vi "MAIN.vi"() -> ()   [LabVIEW 2016, in "副屏.lvlib"]
uses:
  <vilib>/Utility/miscctls.llb/LVPointTypeDef.ctl
  PLC/PLC.lvlib
  <vilib>/Utility/config.llb/NI_LVConfig.lvlib
panel:
  out "单位":string
  out "测试浓度":string
  out "英文标题":string
  out "中文标题":string
  out "公司名称":string
  out "时间":string="2018"
  out "日":string="12"
  out "月":string="12"
  out "年":string="2018"
  # "年"
  # "月"
  # "日"
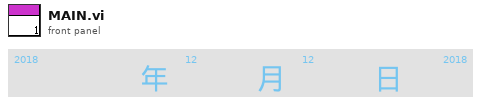
[diagram p1: front panel]
types:
  T1 = cluster{"显示参数中文名":string, "显示参数英文名":string, "显示浓度":string, "显示单位":string}
  T2 = typedef "LVPointTypeDef.ctl" = cluster{"Horizontal":i16, "Vertical":i16}
  T3 = typedef "NI_LVConfig.lvlib/Config Data RefNum.ctl" = refnum<k1>
  T4 = cluster{"AD0":sgl, "AD1":sgl, "AD2":sgl, "AD3":sgl, "AD4":sgl, "AD5":sgl}
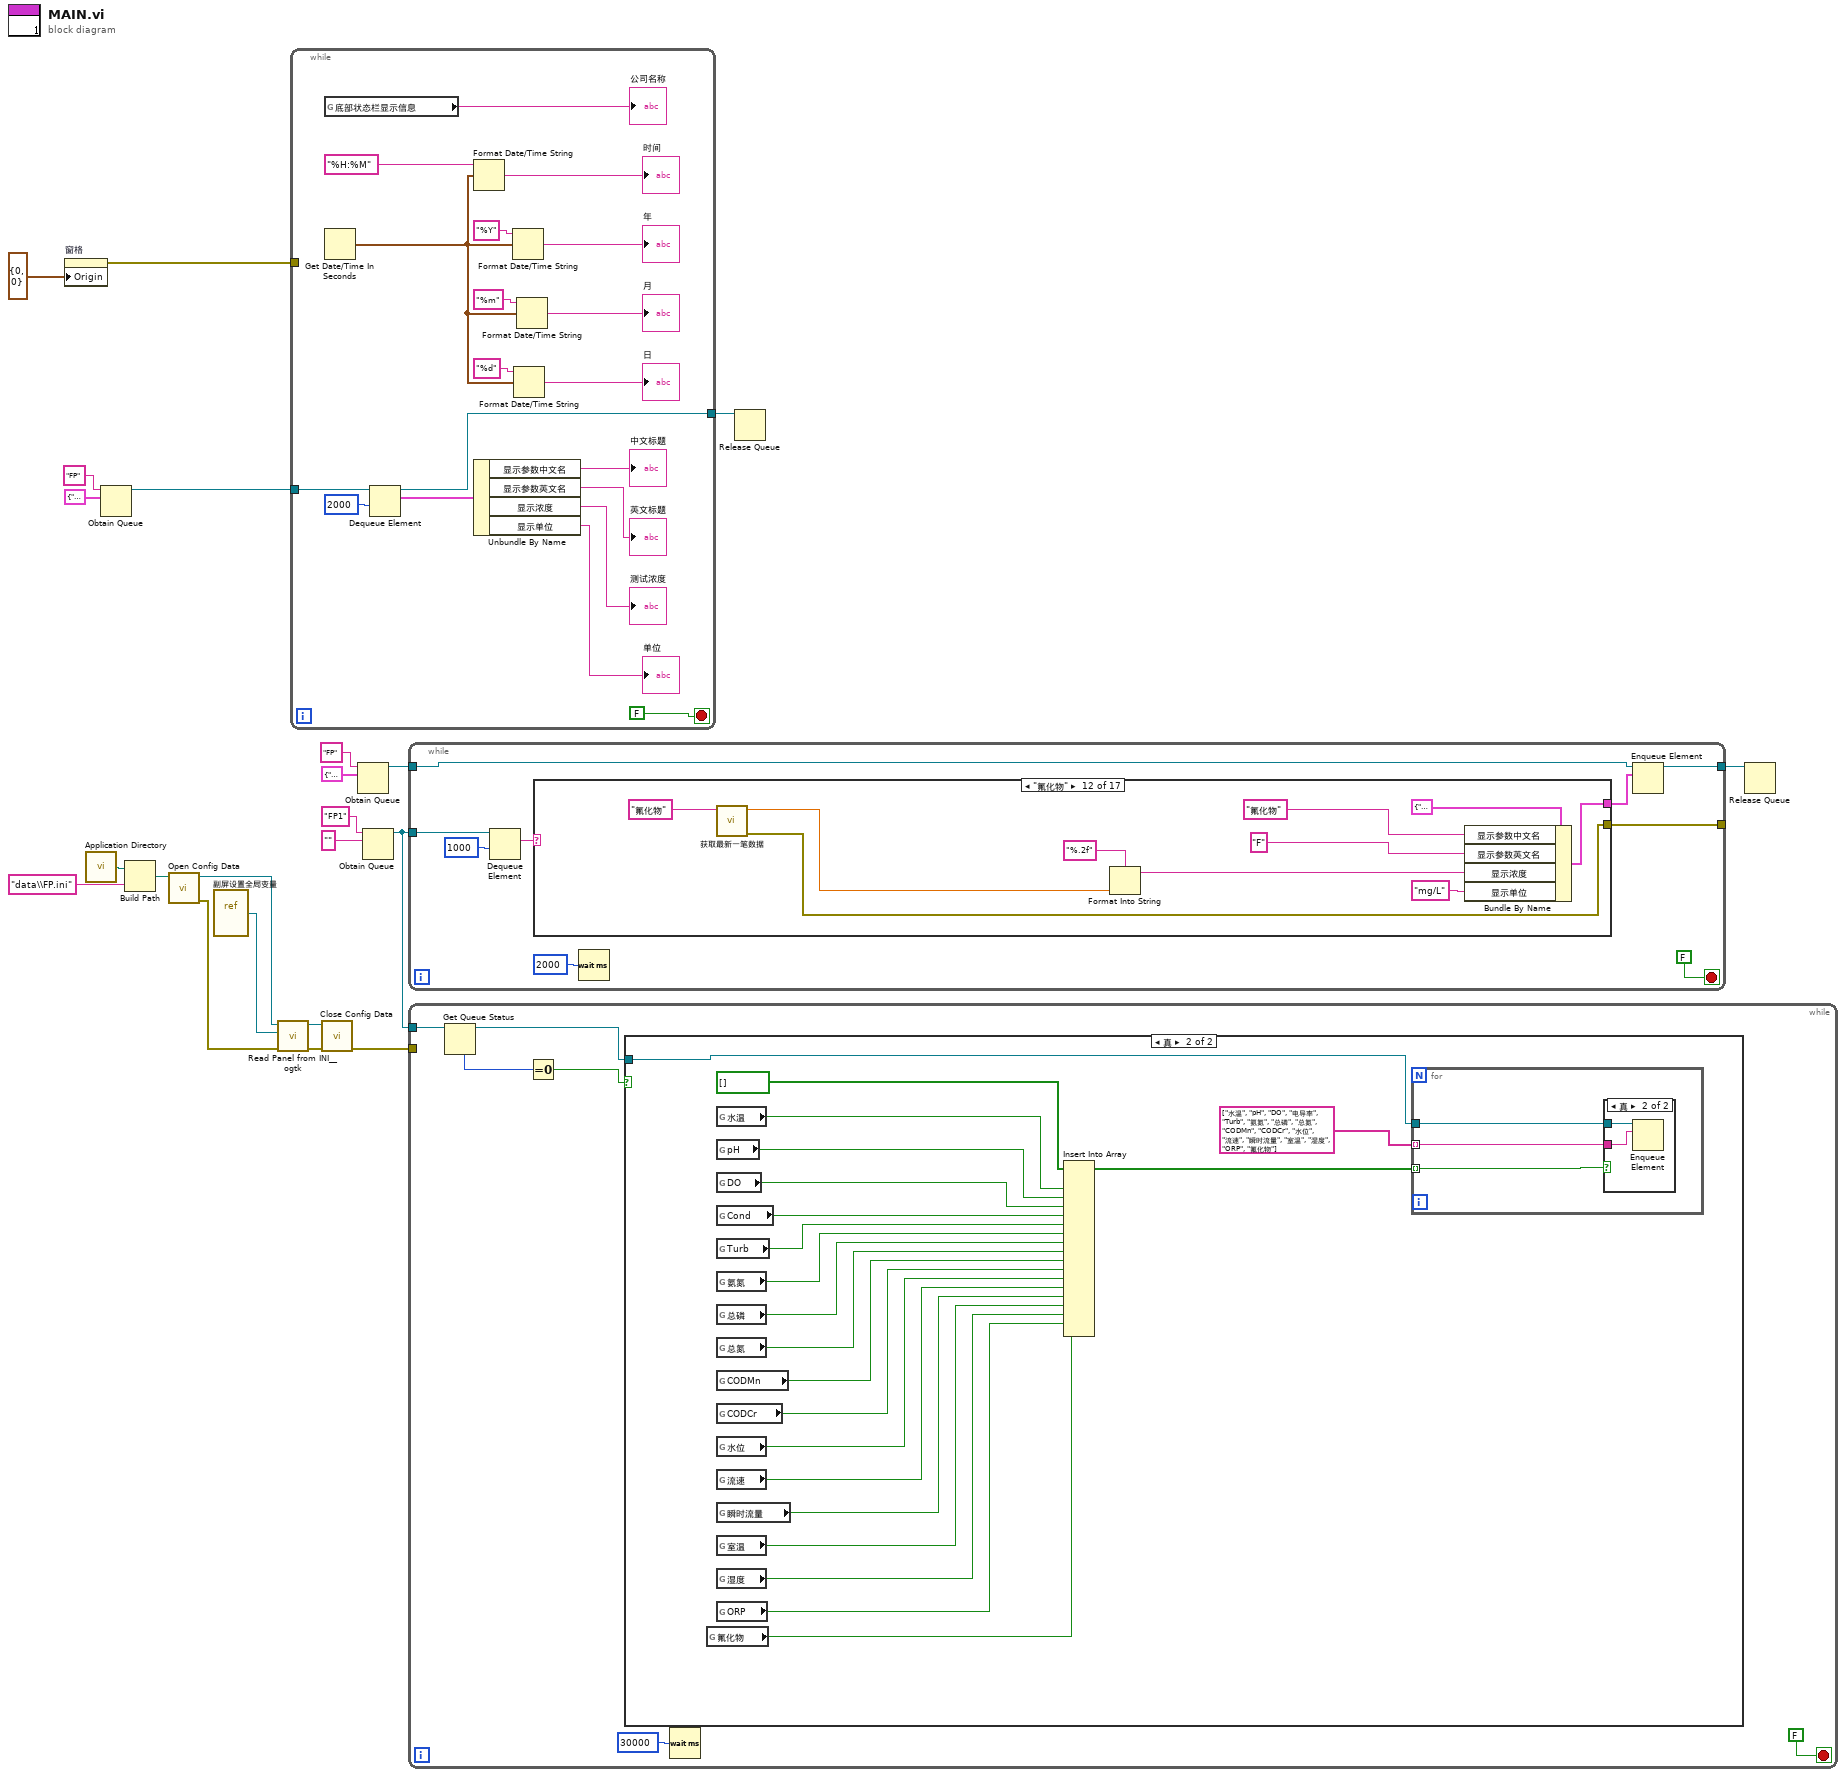
[diagram p0: block diagram]
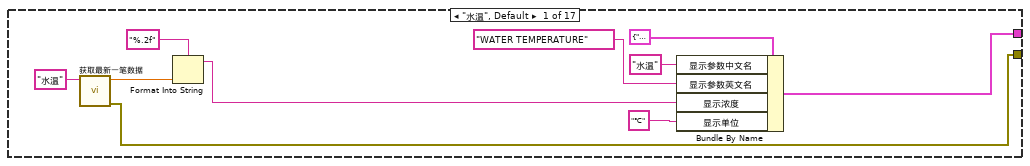
[diagram p4: hidden frame]
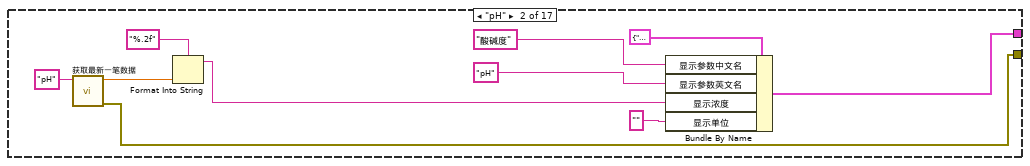
[diagram p5: hidden frame]
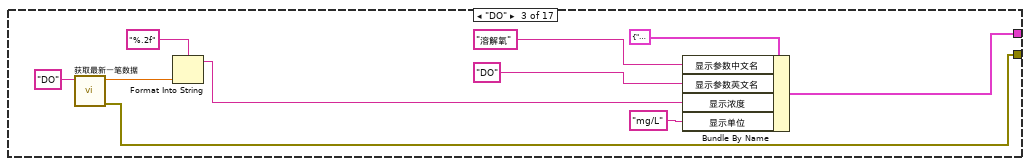
[diagram p6: hidden frame]
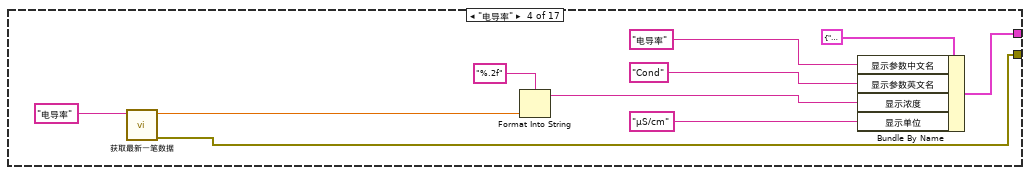
[diagram p7: hidden frame]
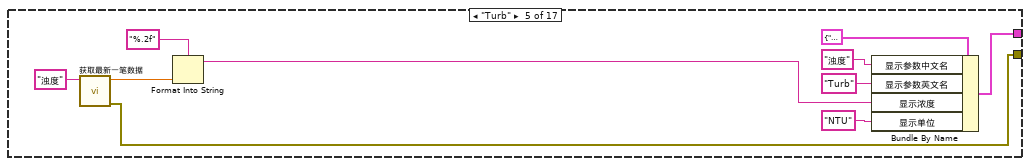
[diagram p8: hidden frame]
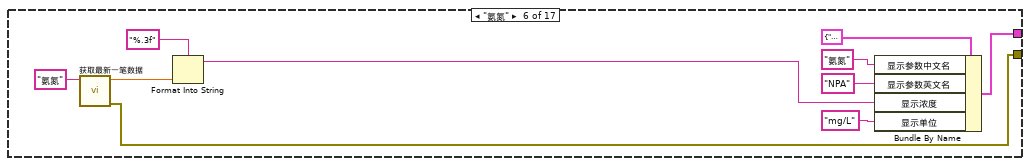
[diagram p9: hidden frame]
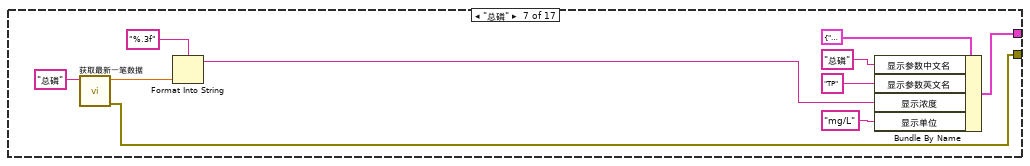
[diagram p10: hidden frame]
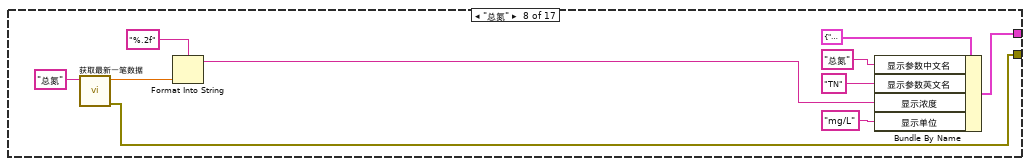
[diagram p11: hidden frame]
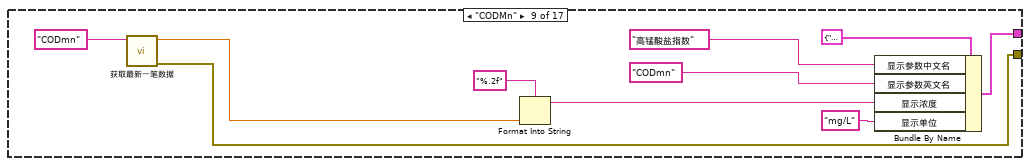
[diagram p12: hidden frame]
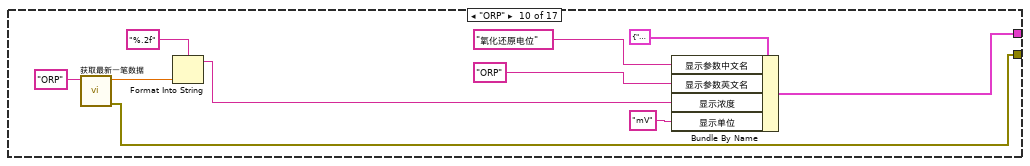
[diagram p13: hidden frame]
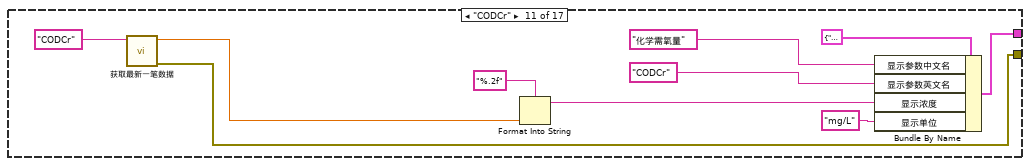
[diagram p14: hidden frame]
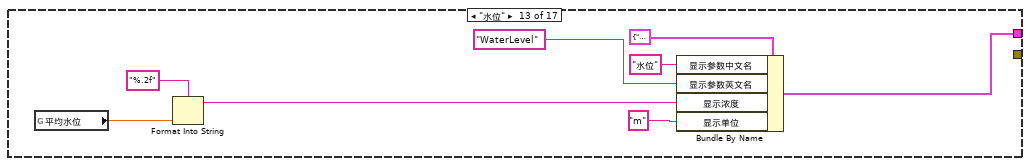
[diagram p15: hidden frame]
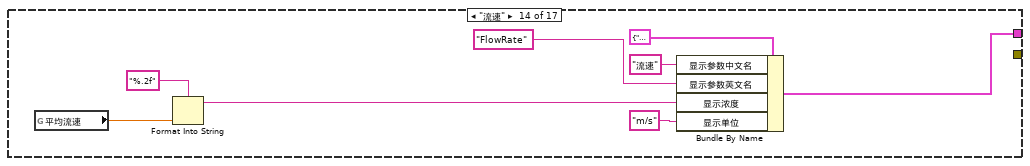
[diagram p16: hidden frame]
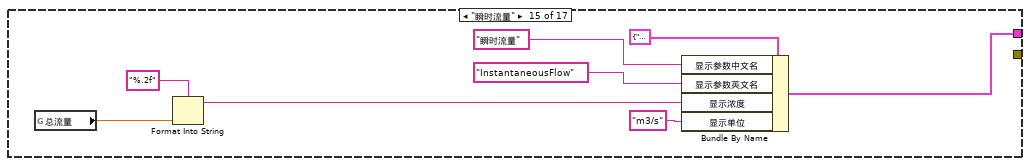
[diagram p17: hidden frame]
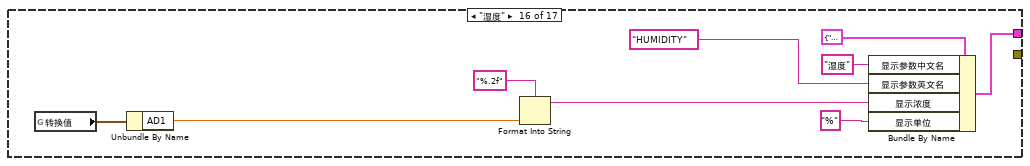
[diagram p18: hidden frame]
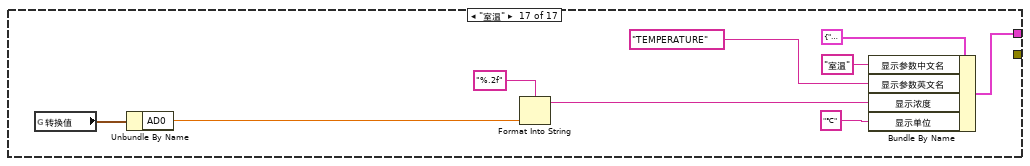
[diagram p19: hidden frame]
diagram:
  n1 = property on="窗格" class="Pane"("Origin"=T2 {"Horizontal"=0, "Vertical"=0} ("原点")) -> (error out=w21:errorcluster)  [unwired: 2 in, 1 out]
  n2 = call <vilib>:"Application Directory.vi"() -> ("Application Directory"=w9:path)
  n3 = Obtain Queue(name (unnamed)="FP" ("名称（未命名）"), element data type=T1 {"显示参数中文名"="", "显示参数英文名"="", "显示浓度"="", "显示单位"=""}) -> (queue out=w18:refnum<queue>)  [unwired: 3 in, 2 out]
  n4 = Build Path(base path=w9, name or relative path="data\\FP.ini" ("名称或相对路径")) -> (appended path=w7:path)
  n5 = call <vilib>:"Open Config Data.vi"("configuration file path"=w7) -> ("error out"=w5:errorcluster, "refnum"=w2:T3)  [unwired: 8 in, 1 out]
  n6 = vi-ref "副屏设置全局变量.vi"() -> (w3:refnum<vi>)
  n7 = call <userlib>:"Read Panel from INI__ogtk.vi"("error in (no error)"=w5, "VI ref"=w3, "refnum"=w2) -> ("error out"=w4:errorcluster, "refnum out"=w1:T3)  [unwired: 7 in]
  n8 = while {
    tunnel: w21 -> [_]
    tunnel: w18 -> [w27]
    tunnel: [w25] -> w17
    stop <- FALSE stop-if-true
    n9 = global read "副屏设置全局变量.vi" "底部状态栏显示信息"() -> (→"公司名称":string)
    n10 = Get Date/Time In Seconds() -> (seconds since 1Jan1904=w33:timestamp)
    n11 = Dequeue Element(queue=w27, timeout in ms (-1)=2000 ("超时毫秒(-1)")) -> (queue out=w25:refnum<queue>, element=w26:T1)  [unwired: 1 in, 2 out]
    n12 = Format Date/Time String(time format string (%c)="%H:%M" ("时间格式字符串(%c)"), seconds (now)=w33) -> (date/time string=→"时间":string)  [unwired: 1 in]
    n13 = Unbundle By Name(w26) -> ("显示参数中文名"=→"中文标题":string, "显示参数英文名"=→"英文标题":string, "显示浓度"=→"测试浓度":string, "显示单位"=→"单位":string)
    n14 = Format Date/Time String(time format string (%c)="%Y" ("时间格式字符串(%c)"), seconds (now)=w33) -> (date/time string=→"年":string)  [unwired: 1 in]
    n15 = Format Date/Time String(time format string (%c)="%d" ("时间格式字符串(%c)"), seconds (now)=w33) -> (date/time string=→"日":string)  [unwired: 1 in]
    n16 = Format Date/Time String(time format string (%c)="%m" ("时间格式字符串(%c)"), seconds (now)=w33) -> (date/time string=→"月":string)  [unwired: 1 in]
  }
  n17 = call <vilib>:"Close Config Data.vi"("error in (no error)"=w4, "refnum"=w1) -> ("error out"=w6:errorcluster)  [unwired: 8 in, 1 out]
  n18 = Obtain Queue(name (unnamed)="FP" ("名称（未命名）"), element data type=T1 {"显示参数中文名"="", "显示参数英文名"="", "显示浓度"="", "显示单位"=""}) -> (queue out=w14:refnum<queue>)  [unwired: 3 in, 2 out]
  n19 = Obtain Queue(name (unnamed)="FP1" ("名称（未命名）"), element data type="") -> (queue out=w10:refnum<queue>)  [unwired: 3 in, 2 out]
  n20 = while {
    tunnel: w14 -> [w50]
    tunnel: [w49] -> w13
    tunnel: [w45] -> _
    tunnel: w10 -> [w44]
    stop <- FALSE stop-if-true
    n21 = Dequeue Element(queue=w44, timeout in ms (-1)=1000 ("超时毫秒(-1)")) -> (element=w42:string)  [unwired: 1 in, 3 out]
    n22 = case shown="\"氟化物\"" w42 {
      tunnel: [w56 w66 w76 w86 w96 w106 w116 w126 w136 w146 w156 w166 w174 w182 w190 w199 w208] -> w46
      tunnel: [w53 w63 w73 w83 w93 w103 w113 w123 w133 w143 w153 w163 _ _ _ _ _] -> w45
      frame "水温", Default {
        n23 = call "获取最新一笔数据.vi"("table"="水温") -> ("错误输出"=w53:errorcluster, "data"=w52:dbl)  [unwired: 8 in, 1 out]
        n24 = Format Into String(format string="%.2f" ("格式字符串"), w52) -> (resulting string=w54:string)  [unwired: 2 in, 1 out]
        n25 = Bundle By Name(cluster=T1 {"显示参数中文名"="", "显示参数英文名"="", "显示浓度"="", "显示单位"=""} ("元素"), "显示参数中文名"="水温", "显示参数英文名"="WATER TEMPERATURE", "显示浓度"=w54, "显示单位"="℃") -> (w56:T1)
      }
      frame "pH" {
        n26 = call "获取最新一笔数据.vi"("table"="pH") -> ("错误输出"=w63:errorcluster, "data"=w61:dbl)  [unwired: 8 in, 1 out]
        n27 = Format Into String(format string="%.2f" ("格式字符串"), w61) -> (resulting string=w64:string)  [unwired: 2 in, 1 out]
        n28 = Bundle By Name(cluster=T1 {"显示参数中文名"="", "显示参数英文名"="", "显示浓度"="", "显示单位"=""} ("元素"), "显示参数中文名"="酸碱度", "显示参数英文名"="pH", "显示浓度"=w64, "显示单位"="") -> (w66:T1)
      }
      frame "DO" {
        n29 = call "获取最新一笔数据.vi"("table"="DO") -> ("错误输出"=w73:errorcluster, "data"=w71:dbl)  [unwired: 8 in, 1 out]
        n30 = Format Into String(format string="%.2f" ("格式字符串"), w71) -> (resulting string=w74:string)  [unwired: 2 in, 1 out]
        n31 = Bundle By Name(cluster=T1 {"显示参数中文名"="", "显示参数英文名"="", "显示浓度"="", "显示单位"=""} ("元素"), "显示参数中文名"="溶解氧", "显示参数英文名"="DO", "显示浓度"=w74, "显示单位"="mg/L") -> (w76:T1)
      }
      frame "电导率" {
        n32 = call "获取最新一笔数据.vi"("table"="电导率") -> ("错误输出"=w83:errorcluster, "data"=w81:dbl)  [unwired: 8 in, 1 out]
        n33 = Format Into String(format string="%.2f" ("格式字符串"), w81) -> (resulting string=w84:string)  [unwired: 2 in, 1 out]
        n34 = Bundle By Name(cluster=T1 {"显示参数中文名"="", "显示参数英文名"="", "显示浓度"="", "显示单位"=""} ("元素"), "显示参数中文名"="电导率", "显示参数英文名"="Cond", "显示浓度"=w84, "显示单位"="μS/cm") -> (w86:T1)
      }
      frame "Turb" {
        n35 = call "获取最新一笔数据.vi"("table"="浊度") -> ("错误输出"=w93:errorcluster, "data"=w91:dbl)  [unwired: 8 in, 1 out]
        n36 = Format Into String(format string="%.2f" ("格式字符串"), w91) -> (resulting string=w94:string)  [unwired: 2 in, 1 out]
        n37 = Bundle By Name(cluster=T1 {"显示参数中文名"="", "显示参数英文名"="", "显示浓度"="", "显示单位"=""} ("元素"), "显示参数中文名"="浊度", "显示参数英文名"="Turb", "显示浓度"=w94, "显示单位"="NTU") -> (w96:T1)
      }
      frame "氨氮" {
        n38 = call "获取最新一笔数据.vi"("table"="氨氮") -> ("错误输出"=w103:errorcluster, "data"=w101:dbl)  [unwired: 8 in, 1 out]
        n39 = Format Into String(format string="%.3f" ("格式字符串"), w101) -> (resulting string=w104:string)  [unwired: 2 in, 1 out]
        n40 = Bundle By Name(cluster=T1 {"显示参数中文名"="", "显示参数英文名"="", "显示浓度"="", "显示单位"=""} ("元素"), "显示参数中文名"="氨氮", "显示参数英文名"="NPA", "显示浓度"=w104, "显示单位"="mg/L") -> (w106:T1)
      }
      frame "总磷" {
        n41 = call "获取最新一笔数据.vi"("table"="总磷") -> ("错误输出"=w113:errorcluster, "data"=w111:dbl)  [unwired: 8 in, 1 out]
        n42 = Format Into String(format string="%.3f" ("格式字符串"), w111) -> (resulting string=w114:string)  [unwired: 2 in, 1 out]
        n43 = Bundle By Name(cluster=T1 {"显示参数中文名"="", "显示参数英文名"="", "显示浓度"="", "显示单位"=""} ("元素"), "显示参数中文名"="总磷", "显示参数英文名"="TP", "显示浓度"=w114, "显示单位"="mg/L") -> (w116:T1)
      }
      frame "总氮" {
        n44 = call "获取最新一笔数据.vi"("table"="总氮") -> ("错误输出"=w123:errorcluster, "data"=w121:dbl)  [unwired: 8 in, 1 out]
        n45 = Format Into String(format string="%.2f" ("格式字符串"), w121) -> (resulting string=w124:string)  [unwired: 2 in, 1 out]
        n46 = Bundle By Name(cluster=T1 {"显示参数中文名"="", "显示参数英文名"="", "显示浓度"="", "显示单位"=""} ("元素"), "显示参数中文名"="总氮", "显示参数英文名"="TN", "显示浓度"=w124, "显示单位"="mg/L") -> (w126:T1)
      }
      frame "CODMn" {
        n47 = call "获取最新一笔数据.vi"("table"="CODmn") -> ("错误输出"=w133:errorcluster, "data"=w132:dbl)  [unwired: 8 in, 1 out]
        n48 = Format Into String(format string="%.2f" ("格式字符串"), w132) -> (resulting string=w134:string)  [unwired: 2 in, 1 out]
        n49 = Bundle By Name(cluster=T1 {"显示参数中文名"="", "显示参数英文名"="", "显示浓度"="", "显示单位"=""} ("元素"), "显示参数中文名"="高锰酸盐指数", "显示参数英文名"="CODmn", "显示浓度"=w134, "显示单位"="mg/L") -> (w136:T1)
      }
      frame "ORP" {
        n50 = call "获取最新一笔数据.vi"("table"="ORP") -> ("错误输出"=w143:errorcluster, "data"=w142:dbl)  [unwired: 8 in, 1 out]
        n51 = Format Into String(format string="%.2f" ("格式字符串"), w142) -> (resulting string=w144:string)  [unwired: 2 in, 1 out]
        n52 = Bundle By Name(cluster=T1 {"显示参数中文名"="", "显示参数英文名"="", "显示浓度"="", "显示单位"=""} ("元素"), "显示参数中文名"="氧化还原电位", "显示参数英文名"="ORP", "显示浓度"=w144, "显示单位"="mV") -> (w146:T1)
      }
      frame "CODCr" {
        n53 = call "获取最新一笔数据.vi"("table"="CODCr") -> ("错误输出"=w153:errorcluster, "data"=w151:dbl)  [unwired: 8 in, 1 out]
        n54 = Format Into String(format string="%.2f" ("格式字符串"), w151) -> (resulting string=w154:string)  [unwired: 2 in, 1 out]
        n55 = Bundle By Name(cluster=T1 {"显示参数中文名"="", "显示参数英文名"="", "显示浓度"="", "显示单位"=""} ("元素"), "显示参数中文名"="化学需氧量", "显示参数英文名"="CODCr", "显示浓度"=w154, "显示单位"="mg/L") -> (w156:T1)
      }
      frame "氟化物" {
        n56 = call "获取最新一笔数据.vi"("table"="氟化物") -> ("错误输出"=w163:errorcluster, "data"=w161:dbl)  [unwired: 8 in, 1 out]
        n57 = Format Into String(format string="%.2f" ("格式字符串"), w161) -> (resulting string=w164:string)  [unwired: 2 in, 1 out]
        n58 = Bundle By Name(cluster=T1 {"显示参数中文名"="", "显示参数英文名"="", "显示浓度"="", "显示单位"=""} ("元素"), "显示参数中文名"="氟化物", "显示参数英文名"="F", "显示浓度"=w164, "显示单位"="mg/L") -> (w166:T1)
      }
      frame "水位" {
        n59 = global read "流量计全局变量.vi" "平均水位"() -> (w171:dbl)
        n60 = Format Into String(format string="%.2f" ("格式字符串"), w171) -> (resulting string=w172:string)  [unwired: 2 in, 1 out]
        n61 = Bundle By Name(cluster=T1 {"显示参数中文名"="", "显示参数英文名"="", "显示浓度"="", "显示单位"=""} ("元素"), "显示参数中文名"="水位", "显示参数英文名"="WaterLevel", "显示浓度"=w172, "显示单位"="m") -> (w174:T1)
      }
      frame "流速" {
        n62 = global read "流量计全局变量.vi" "平均流速"() -> (w179:dbl)
        n63 = Format Into String(format string="%.2f" ("格式字符串"), w179) -> (resulting string=w180:string)  [unwired: 2 in, 1 out]
        n64 = Bundle By Name(cluster=T1 {"显示参数中文名"="", "显示参数英文名"="", "显示浓度"="", "显示单位"=""} ("元素"), "显示参数中文名"="流速", "显示参数英文名"="FlowRate", "显示浓度"=w180, "显示单位"="m/s") -> (w182:T1)
      }
      frame "瞬时流量" {
        n65 = global read "流量计全局变量.vi" "总流量"() -> (w187:dbl)
        n66 = Format Into String(format string="%.2f" ("格式字符串"), w187) -> (resulting string=w188:string)  [unwired: 2 in, 1 out]
        n67 = Bundle By Name(cluster=T1 {"显示参数中文名"="", "显示参数英文名"="", "显示浓度"="", "显示单位"=""} ("元素"), "显示参数中文名"="瞬时流量", "显示参数英文名"="InstantaneousFlow", "显示浓度"=w188, "显示单位"="m3/s") -> (w190:T1)
      }
      frame "湿度" {
        n68 = global read "采配水全局变量.vi" "转换值"() -> (w196:T4)
        n69 = Unbundle By Name(w196) -> ("AD1"=w198:sgl)
        n70 = Format Into String(format string="%.2f" ("格式字符串"), w198) -> (resulting string=w195:string)  [unwired: 2 in, 1 out]
        n71 = Bundle By Name(cluster=T1 {"显示参数中文名"="", "显示参数英文名"="", "显示浓度"="", "显示单位"=""} ("元素"), "显示参数中文名"="湿度", "显示参数英文名"="HUMIDITY", "显示浓度"=w195, "显示单位"="%") -> (w199:T1)
      }
      frame "室温" {
        n72 = global read "采配水全局变量.vi" "转换值"() -> (w205:T4)
        n73 = Unbundle By Name(w205) -> ("AD0"=w207:sgl)
        n74 = Format Into String(format string="%.2f" ("格式字符串"), w207) -> (resulting string=w204:string)  [unwired: 2 in, 1 out]
        n75 = Bundle By Name(cluster=T1 {"显示参数中文名"="", "显示参数英文名"="", "显示浓度"="", "显示单位"=""} ("元素"), "显示参数中文名"="室温", "显示参数英文名"="TEMPERATURE", "显示浓度"=w204, "显示单位"="℃") -> (w208:T1)
      }
    }
    n76 = Wait (ms)(milliseconds to wait=u32 2000 ("等待时间（毫秒）")) -> ()  [unwired: 1 out]
    n77 = Enqueue Element(queue=w50, element=w46) -> (queue out=w49:refnum<queue>)  [unwired: 2 in, 2 out]
  }
  n78 = while {
    tunnel: w10 -> [w217]
    tunnel: w6 -> [_]
    stop <- FALSE stop-if-true
    n79 = Get Queue Status(queue=w217) -> (queue out=w214:refnum<queue>, # elements in queue=w216:i32)  [unwired: 2 in, 6 out]
    n80 = Equal To 0?(x=w216) -> (x = 0?=w215:bool)
    n81 = case shown="真" w215 {
      tunnel: w214 -> [_ w239]
      frame False {
      }
      frame True {
        n82 = global read "副屏设置全局变量.vi" "氟化物"() -> (w219:bool)
        n83 = global read "副屏设置全局变量.vi" "水温"() -> (w237:bool)
        n84 = global read "副屏设置全局变量.vi" "pH"() -> (w236:bool)
        n85 = global read "副屏设置全局变量.vi" "DO"() -> (w235:bool)
        n86 = global read "副屏设置全局变量.vi" "Cond"() -> (w234:bool)
        n87 = global read "副屏设置全局变量.vi" "Turb"() -> (w233:bool)
        n88 = global read "副屏设置全局变量.vi" "氨氮"() -> (w232:bool)
        n89 = global read "副屏设置全局变量.vi" "总磷"() -> (w231:bool)
        n90 = global read "副屏设置全局变量.vi" "总氮"() -> (w230:bool)
        n91 = global read "副屏设置全局变量.vi" "CODMn"() -> (w229:bool)
        n92 = global read "副屏设置全局变量.vi" "CODCr"() -> (w228:bool)
        n93 = global read "副屏设置全局变量.vi" "水位"() -> (w227:bool)
        n94 = global read "副屏设置全局变量.vi" "流速"() -> (w226:bool)
        n95 = global read "副屏设置全局变量.vi" "瞬时流量"() -> (w225:bool)
        n96 = global read "副屏设置全局变量.vi" "室温"() -> (w224:bool)
        n97 = global read "副屏设置全局变量.vi" "湿度"() -> (w223:bool)
        n98 = global read "副屏设置全局变量.vi" "ORP"() -> (w220:bool)
        n99 = Insert Into Array(array=bool[] [], new element #1=w237, new element #2=w236, new element #3=w235, new element #4=w234, new element #5=w233, new element #6=w232, new element #7=w231, new element #8=w230, new element #9=w229, new element #10=w228, new element #11=w227, new element #12=w226, new element #13=w225, new element #14=w224, new element #15=w223, new element #16=w220, new element #17=w219) -> (w222:bool[])  [unwired: 1 in]
        n100 = for {
          tunnel: w239 -> [w242]
          tunnel: w222 -> [w241] mode=indexing
          tunnel: string[] ["水温", "pH", "DO", "电导率", "Turb", "氨氮", "总磷", "总氮", "CODMn", "CODCr", "水位", "流速", "瞬时流量", "室温", "湿度", "ORP", "氟化物"] -> [w240] mode=indexing
          n101 = case shown="真" w241 {
            tunnel: w242 -> [_ w244]
            tunnel: w240 -> [_ w243]
            frame False {
            }
            frame True {
              n102 = Enqueue Element(queue=w244, element=w243) -> ()  [unwired: 2 in, 3 out]
            }
          }
        }
      }
    }
    n103 = Wait (ms)(milliseconds to wait=u32 30000 ("等待时间（毫秒）")) -> ()  [unwired: 1 out]
  }
  n104 = Release Queue(queue=w17) -> ()  [unwired: 2 in, 3 out]
  n105 = Release Queue(queue=w13) -> ()  [unwired: 2 in, 3 out]
